vi "Step Convert Test Record To jsRecord.vi"(3 "Test Record":T2) -> (1 "STEP jsRecord":T1)   [LabVIEW 2011]
uses:
  Tests/Test Record.ctl
  Step jsRecord.ctl
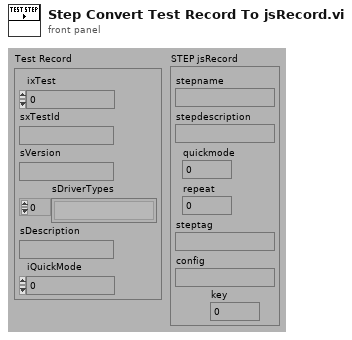
[diagram p1: front panel]
types:
  T1 = typedef "STEP jsRecord.ctl" = cluster{"stepname":string, "stepdescription":string, "quickmode":i32, "repeat":i32, "steptag":string, "config":string, "key":i32}
  T2 = typedef "Test Record.ctl" = cluster{"ixTest":i32, "sxTestId":string, "sVersion":string, "sDriverTypes":string[], "sDescription":string, "iQuickMode":i32}
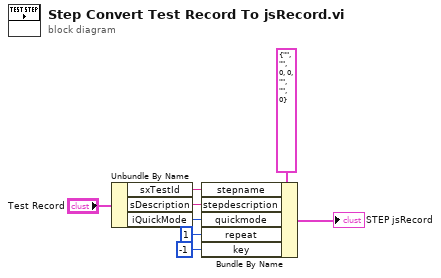
[diagram p0: block diagram]
diagram:
  n1 = Unbundle By Name("Test Record") -> ("sxTestId"=w7:string, "sDescription"=w6:string, "iQuickMode"=w5:i32)
  n2 = Bundle By Name(cluster=T1 {"stepname"="", "stepdescription"="", "quickmode"=0, "repeat"=0, "steptag"="", "config"="", "key"=0} ("STEP jsRecord"), "stepname"=w7, "stepdescription"=w6, "quickmode"=w5, "repeat"=1 ("config"), "key"=-1 ("config")) -> (→"STEP jsRecord":T1)
